vi "New Panel GUI Manager.vi"(8 "error in (no error)":errorcluster, 11 "Panel GUI Manager in":refnum<class "Panel GUI Manager.lvclass">) -> (0 "error out":errorcluster, 3 "Panel GUI Manager out":refnum<class "Panel GUI Manager.lvclass">)   [LabVIEW 2015, in "Panel GUI Manager.lvclass"]
uses:
  Panel GUI Manager.lvclass
  GUI/GUI Controls/GUI Control/GUI Control.lvclass
  Panel GUI Manager.lvclass/Panel GUI Manager.ctl
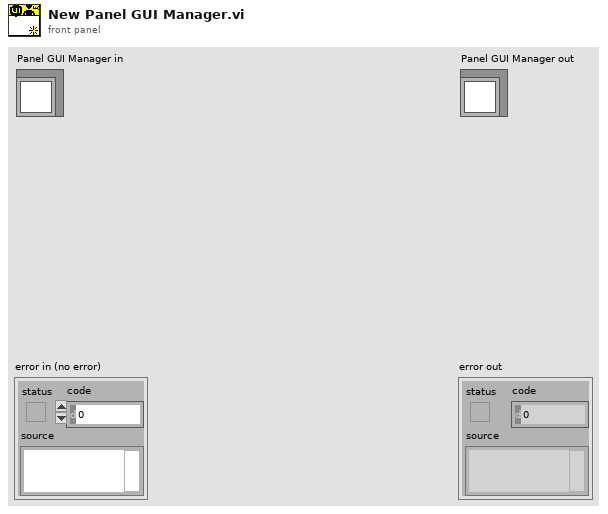
[diagram p1: front panel]
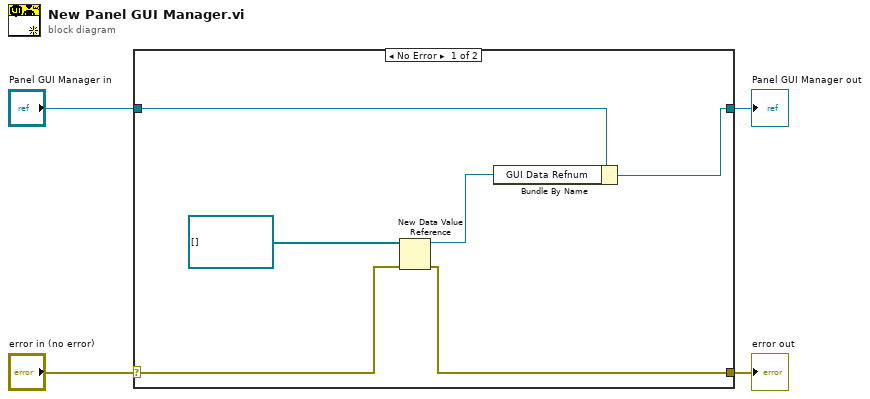
[diagram p0: block diagram]
diagram:
  n1 = case shown="No Error" "error in (no error)" {
    selector: "error in (no error)" -> [w8 w12]
    tunnel: [w6 w12] -> w3
    tunnel: [w5 w11] -> w1
    tunnel: "Panel GUI Manager in" -> [w9 w11]
    frame No Error {
      n2 = New Data Value Reference(data value=refnum<class "GUI Control.lvclass">[] [] ("Gui Controls_Class"), error in=w8) -> (data value reference=w7:refnum<data-value>, error out=w6:errorcluster)
      n3 = Bundle By Name(cluster=w9, "GUI Data Refnum"=w7) -> (w5:refnum<class "Panel GUI Manager.lvclass">)
    }
    frame Error {
    }
  }
  "error out" <- w3
  "Panel GUI Manager out" <- w1
